vi "Get SubVI Ref QD.vi"(8 "error in (no error)":errorcluster, 11 "Affected Items":T1) -> (0 "error out":errorcluster, 3 "Selected SubVI Reference":refnum<vi>)   [LabVIEW 2017]
doc: "Returns the VI reference of the selected SubVI."
uses:
  plugins/PopupMenus/edit time panel and diagram/Open DQMH Request Message Diagram.llb/Open DQMH Request Message Diagram.ctl
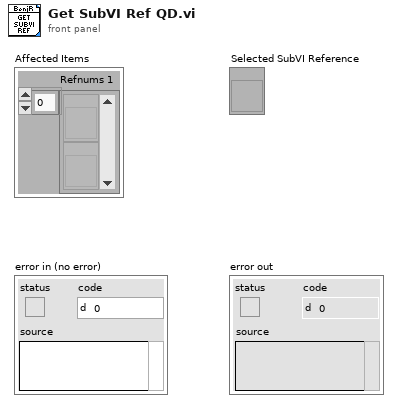
[diagram p1: front panel]
types:
  T1 = typedef "Open DQMH Request Message Diagram.ctl" = cluster{"Refnums 1":refnum<vi>[]}
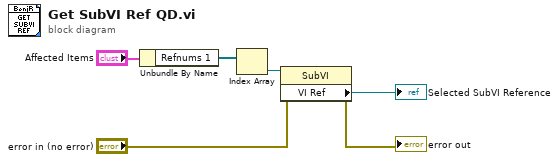
[diagram p0: block diagram]
diagram:
  n1 = Unbundle By Name("Affected Items") -> ("Refnums 1"=w5:refnum<vi>[])
  n2 = Index Array(array=w5) -> (element=w4:refnum<vi>)  [unwired: 1 in]
  n3 = property class="SubVI"(reference=w4, error in="error in (no error)") -> (error out=→"error out":errorcluster, "VI Ref"=→"Selected SubVI Reference":refnum<vi>)  [unwired: 1 out]
